vi "ex3.vi"() -> ()   [LabVIEW 2022 SP3]
uses:
  <vilib>/numeric/Random Number (Range) DBL.vi
panel:
  out "LED":bool
  in  "Loop Delay [ms]":dbl
  in  "?":bool
  in  "Noises Amplitude":dbl
  out "Waveform Chart":cluster{dbl, "Discrimination level":dbl}(graph)
  in  "Discrimination level":dbl
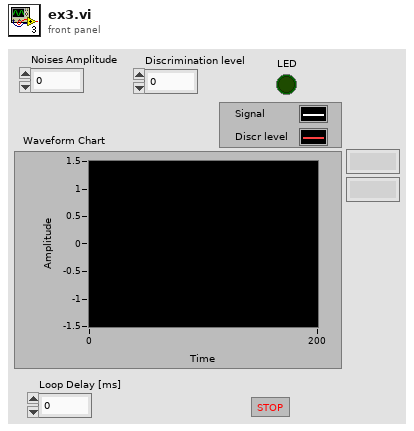
[diagram p1: front panel]
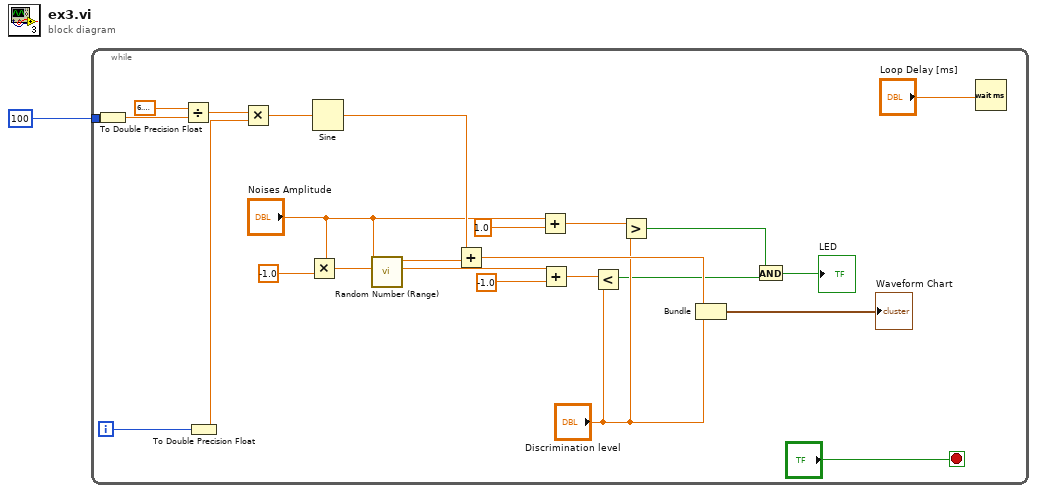
[diagram p0: block diagram]
diagram:
  n1 = while {
    tunnel: 100 -> [w15]
    i -> [w23]
    stop <- "?" stop-if-true
    n2 = To Double Precision Float(number=w15) -> (double precision float=w21:dbl)
    n3 = Divide(x=6.283185307179586, y=w21) -> (x/y=w24:dbl)
    n4 = To Double Precision Float(number=w23) -> (double precision float=w22:dbl)
    n5 = Multiply(x=w24, y=w22) -> (x*y=w18:dbl)
    n6 = Multiply(x="Noises Amplitude", y=-1.0) -> (x*y=w9:dbl)
    n7 = Sine(x=w18) -> (sin(x)=w12:dbl)
    n8 = call-poly <vilib>:"Random Number (Range).vi"("lower bound (0)"=w9, "upper bound (100)"="Noises Amplitude") -> ("number"=w17:dbl)  [unwired: 9 in]
    n9 = Add(x=w12, y=w17) -> (x+y=w16:dbl)
    n10 = Add(x="Noises Amplitude", y=1.0) -> (x+y=w7:dbl)
    n11 = Add(x=w9, y=-1.0) -> (x+y=w6:dbl)
    n12 = Less?(x=w6, y="Discrimination level") -> (x < y?=w3:bool)
    n13 = Greater?(x=w7, y="Discrimination level") -> (0:w4:bool)
    n14 = Bundle(w16, "Discrimination level"="Discrimination level") -> (→"Waveform Chart":cluster{dbl, "Discrimination level":dbl})  [unwired: 1 in]
    n15 = And(x=w4, y=w3) -> (x .and. y?=→"LED":bool)
    n16 = Wait (ms)(milliseconds to wait="Loop Delay [ms]") -> ()  [unwired: 1 out]
  }
